vi "global_var.vi"() -> ()   [LabVIEW 2013]
panel:
  in  "GUI strings":string[](array[string])
  out "nElementsQueue":i32 caption="Elements in Queue"
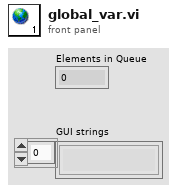
[diagram p1: front panel]
diagram:
